vi "SP Convert 1.0 - 1.2 to 1.3 - 1.4.vi"(1 "S Parameter 1.0 - 1.2 Test Parameters":T2 {"Stimulus"."Sweep Time, s" format="%.3g"}) -> (0 "S Parameter 1.3 - 1.4 Test Parameters":T1 {"Stimulus"."Sweep Time, s" format="%.3g"; "Measurements"."Channel (CH 1)" items=["CH 1", "CH 2", "CH 3", "CH 4"]})   [LabVIEW 2011]
uses:
  TypeDefs/SP Test Parameters v1.0-1.2.ctl
  TypeDefs/SP Test Parameters v1.3-1.4.ctl
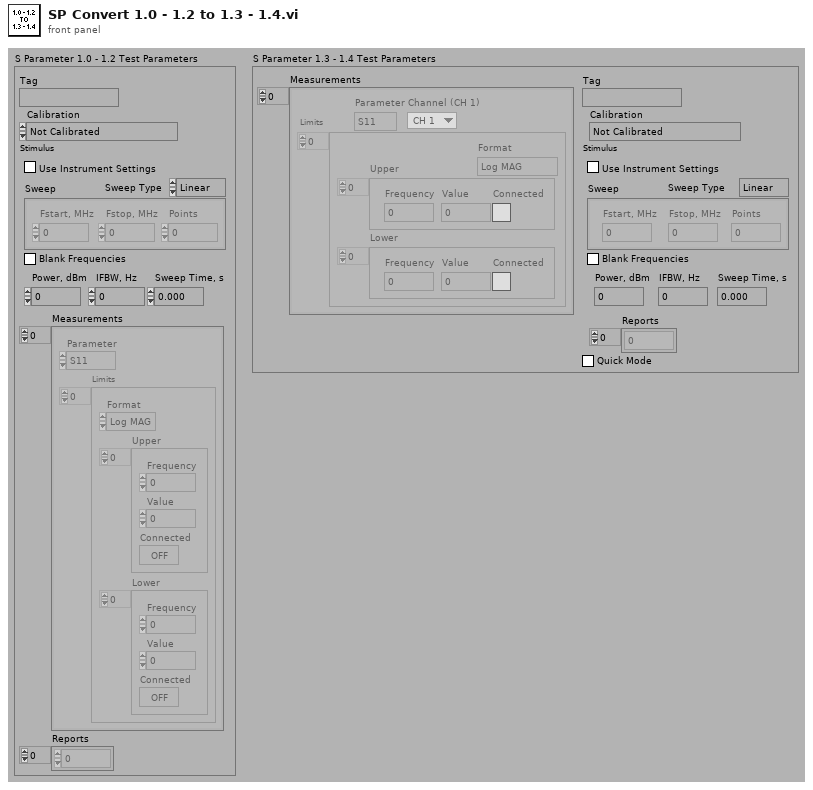
[diagram p1: front panel]
types:
  T1 = typedef "SP Test Parameters v1.3-1.4.ctl" = cluster{"Tag":string, "Calibration":enum32{"Not Calibrated", "Response", "Response and Isolation", "Full 1-Port (Port 1)", "Full 1-Port (Port 2)", "Full 2-Port", "One Path 2-Port", "TRL/LRM  2-Port"}, "Stimulus":cluster{"Use Instrument Settings":bool, "Sweep Type":enum32{"Linear", "Log", "List", "Power", "CW"}, "Sweep":cluster{"Fstart, MHz":dbl, "Fstop, MHz":dbl, "Points":i32}[], "Blank Frequencies":bool, "Power, dBm":dbl, "IFBW, Hz":dbl, "Sweep Time, s":dbl}, "Measurements":cluster{"Parameter":enum32{"S11", "S21", "S12", "S22"}, "Limits":cluster{"Format":enum16{"Log MAG", "Lin MAG", "VSWR", "Phase", "Delay", "Insertion Loss", "Isolation", "Return Loss"}, "Upper":cluster{"Frequency":dbl, "Value":dbl, "Connected":bool}[], "Lower":cluster{"Frequency":dbl, "Value":dbl, "Connected":bool}[]}[], "Channel (CH 1)":u16}[], "Reports":i32[], "Quick Mode":bool}
  T2 = typedef "SP Test Parameters v1.0-1.2.ctl" = cluster{"Tag":string, "Calibration":enum32{"Not Calibrated", "Response", "Response and Isolation", "Full 1-Port (Port 1)", "Full 1-Port (Port 2)", "Full 2-Port"}, "Stimulus":cluster{"Use Instrument Settings":bool, "Sweep Type":enum32{"Linear", "Log", "List", "Power", "CW"}, "Sweep":cluster{"Fstart, MHz":dbl, "Fstop, MHz":dbl, "Points":i32}[], "Blank Frequencies":bool, "Power, dBm":dbl, "IFBW, Hz":dbl, "Sweep Time, s":dbl}, "Measurements":cluster{"Parameter":enum32{"S11", "S21", "S12", "S22"}, "Limits":cluster{"Format":enum16{"Log MAG", "Lin MAG", "VSWR", "Phase", "Delay", "Insertion Loss", "Isolation", "Return Loss"}, "Upper":cluster{"Frequency":dbl, "Value":dbl, "Connected":bool}[], "Lower":cluster{"Frequency":dbl, "Value":dbl, "Connected":bool}[]}[]}[], "Reports":i32[]}
  T3 = enum32{"Not Calibrated", "Response", "Response and Isolation", "Full 1-Port (Port 1)", "Full 1-Port (Port 2)", "Full 2-Port"}
  T4 = cluster{"Use Instrument Settings":bool, "Sweep Type":enum32{"Linear", "Log", "List", "Power", "CW"}, "Sweep":cluster{"Fstart, MHz":dbl, "Fstop, MHz":dbl, "Points":i32}[], "Blank Frequencies":bool, "Power, dBm":dbl, "IFBW, Hz":dbl, "Sweep Time, s":dbl}
  T5 = cluster{"Parameter":enum32{"S11", "S21", "S12", "S22"}, "Limits":cluster{"Format":enum16{"Log MAG", "Lin MAG", "VSWR", "Phase", "Delay", "Insertion Loss", "Isolation", "Return Loss"}, "Upper":cluster{"Frequency":dbl, "Value":dbl, "Connected":bool}[], "Lower":cluster{"Frequency":dbl, "Value":dbl, "Connected":bool}[]}[]}[]
  T6 = cluster{"Parameter":enum32{"S11", "S21", "S12", "S22"}, "Limits":cluster{"Format":enum16{"Log MAG", "Lin MAG", "VSWR", "Phase", "Delay", "Insertion Loss", "Isolation", "Return Loss"}, "Upper":cluster{"Frequency":dbl, "Value":dbl, "Connected":bool}[], "Lower":cluster{"Frequency":dbl, "Value":dbl, "Connected":bool}[]}[], "Channel (CH 1)":u16}[]
  T7 = cluster{"Parameter":enum32{"S11", "S21", "S12", "S22"}, "Limits":cluster{"Format":enum16{"Log MAG", "Lin MAG", "VSWR", "Phase", "Delay", "Insertion Loss", "Isolation", "Return Loss"}, "Upper":cluster{"Frequency":dbl, "Value":dbl, "Connected":bool}[], "Lower":cluster{"Frequency":dbl, "Value":dbl, "Connected":bool}[]}[], "Channel (CH 1)":u16}
  T8 = cluster{"Format":enum16{"Log MAG", "Lin MAG", "VSWR", "Phase", "Delay", "Insertion Loss", "Isolation", "Return Loss"}, "Upper":cluster{"Frequency":dbl, "Value":dbl, "Connected":bool}[], "Lower":cluster{"Frequency":dbl, "Value":dbl, "Connected":bool}[]}[]
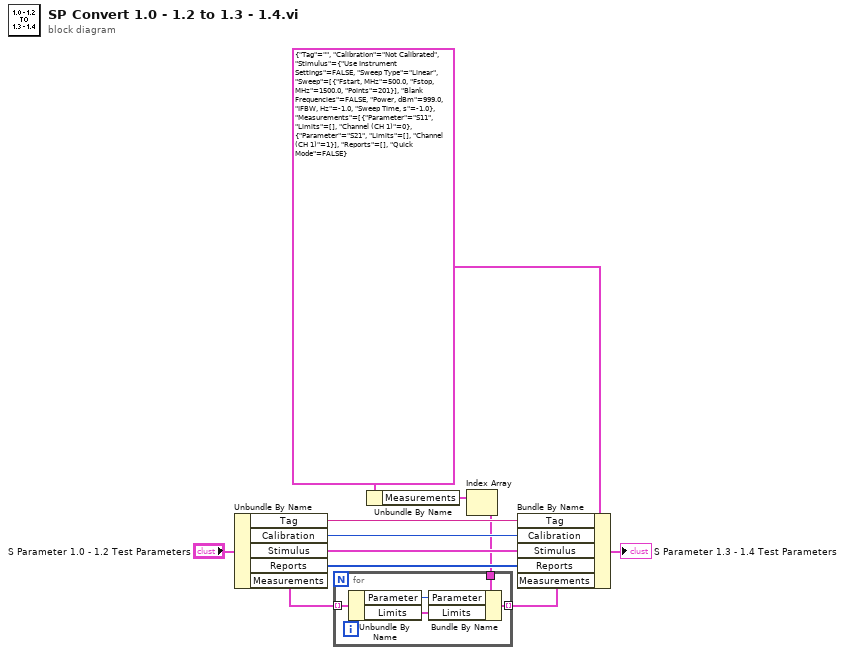
[diagram p0: block diagram]
diagram:
  w5 = T1 {"Tag"="", "Calibration"=enum."Not Calibrated", "Stimulus"={"Use Instrument Settings"=FALSE, "Sweep Type"=enum."Linear", "Sweep"=[{"Fstart, MHz"=500.0, "Fstop, MHz"=1500.0, "Points"=201}], "Blank Frequencies"=FALSE, "Power, dBm"=999.0, "IFBW, Hz"=-1.0, "Sweep Time, s"=-1.0}, "Measurements"=[{"Parameter"=enum."S11", "Limits"=[], "Channel (CH 1)"=0}, {"Parameter"=enum."S21", "Limits"=[], "Channel (CH 1)"=1}], "Reports"=[], "Quick Mode"=FALSE} ("S Parameter Test Parameters")
  n1 = Unbundle By Name("S Parameter 1.0 - 1.2 Test Parameters") -> ("Tag"=w10:string, "Calibration"=w9:T3, "Stimulus"=w8:T4, "Reports"=w7:i32[], "Measurements"=w6:T5)
  n2 = Unbundle By Name(w5) -> ("Measurements"=w4:T6)
  n3 = Index Array(array=w4) -> (element=w3:T7)  [unwired: 1 in]
  n4 = for {
    tunnel: w6 -> [w16] mode=indexing
    tunnel: w3 -> [w15]
    tunnel: [w12] -> w2 mode=indexing
    n5 = Unbundle By Name(w16) -> ("Parameter"=w14:enum32{"S11", "S21", "S12", "S22"}, "Limits"=w13:T8)
    n6 = Bundle By Name(cluster=w15, "Parameter"=w14, "Limits"=w13) -> (w12:T7)
  }
  n7 = Bundle By Name(cluster=w5, "Tag"=w10, "Calibration"=w9, "Stimulus"=w8, "Reports"=w7, "Measurements"=w2) -> (→"S Parameter 1.3 - 1.4 Test Parameters":T1)
